vi "File Read Only.vi"(8 "error in (no error)":errorcluster, 11 "Path in":path) -> (0 "error out":errorcluster, 3 "Path out":path)   [LabVIEW 2018]
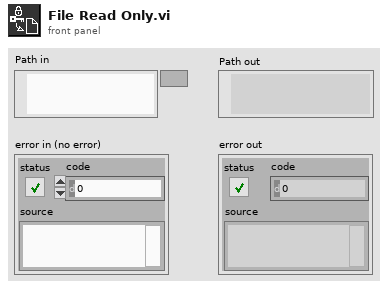
[diagram p1: front panel]
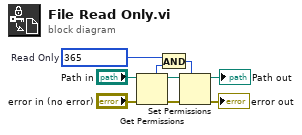
[diagram p0: block diagram]
diagram:
  w7 = i16 365  # Read Only
  n1 = Get Permissions(8:"error in (no error)", 11:"Path in") -> (0:w8:errorcluster, 3:w9:path, 5:w6:i16)  [unwired: 2 out]
  n2 = And(x=w7, y=w6) -> (x .and. y?=w5:i16)
  n3 = Set Permissions(7:w5, 8:w8, 11:w9) -> (0:→"error out":errorcluster, 3:→"Path out":path)  [unwired: 2 in]
